vi "New Star.vi"(8 "error in (no error)":errorcluster, 10 "Board Game in":refnum<class "Board Game.lvclass">, 11 "Star in":refnum<class "Star.lvclass">) -> (0 "error out":errorcluster, 3 "Star out":refnum<class "Star.lvclass">)   [LabVIEW 2021, in "Star.lvclass"]
uses:
  Star.lvclass
  C:/Users/poche/Programs/LabVIEW/imposible snake/GameEl_class/GameEl.lvclass
  Board Game_class/Board Game.lvclass
  GameEl_class/GameEl.lvclass/GameEl.ctl
  Board Game_class/Board Game.lvclass/Board Game.ctl
  Star.lvclass/Star.ctl
  Board Game_class/Read Size.vi
  GameEl_class/GameEl.lvclass
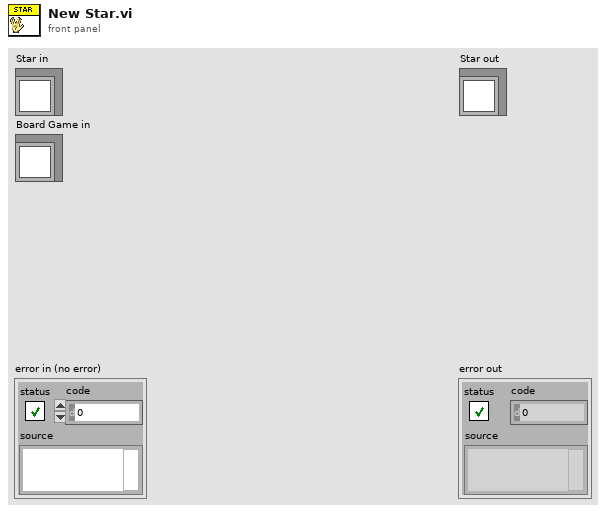
[diagram p1: front panel]
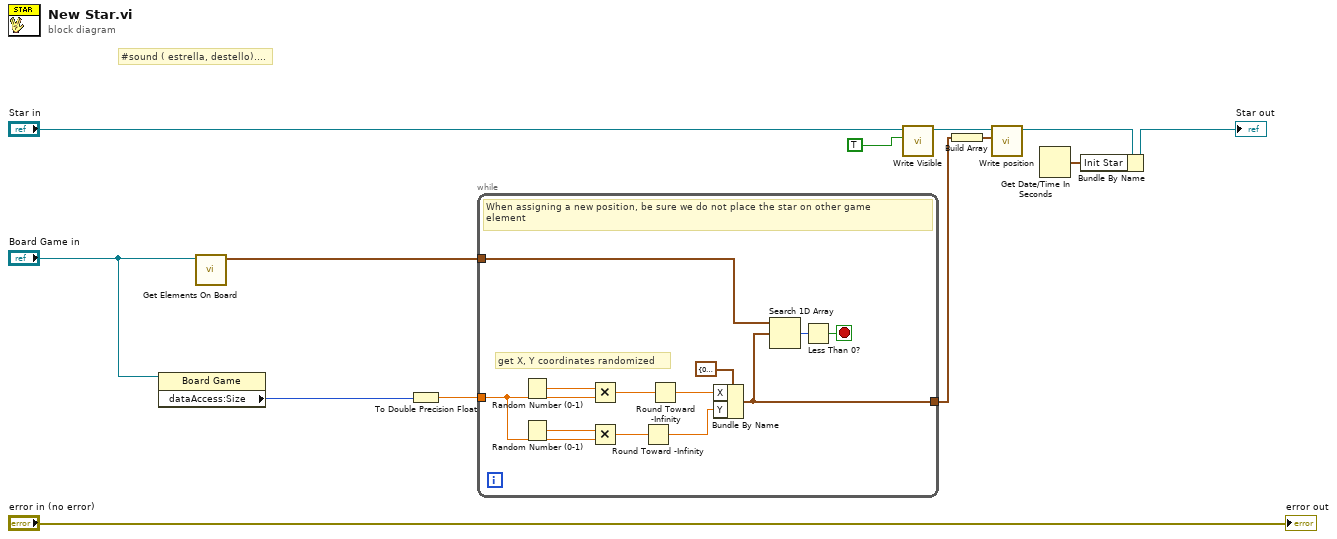
[diagram p0: block diagram]
diagram:
  # "#sound ( estrella, destello)...."
  n1 = property class="Board Game"(reference="Board Game in") -> ("dataAccess:Size"=w10:u16)  [unwired: 1 in, 2 out]
  n2 = call "Get Elements On Board.vi"("Board Game in"="Board Game in") -> ("position"=w2:cluster{"x":dbl, "y":dbl}[])  [unwired: 9 in, 1 out]
  n3 = To Double Precision Float(number=w10) -> (double precision float=w8:dbl)
  n4 = while {
    tunnel: w8 -> [w23]
    tunnel: [w16] -> w5
    tunnel: w2 -> [w15]
    stop <- w14 stop-if-true
    # "get X, Y coordinates randomized"
    # "When assigning a new position, be sure we do not place the star on other game \nelement"
    n5 = Random Number (0-1)() -> (number: 0 to 1=w25:dbl)
    n6 = Random Number (0-1)() -> (number: 0 to 1=w24:dbl)
    n7 = Multiply(x=w25, y=w23) -> (x*y=w21:dbl)
    n8 = Multiply(x=w24, y=w23) -> (x*y=w20:dbl)
    n9 = Round Toward -Infinity(1:w20) -> (0:w17:dbl)
    n10 = Round Toward -Infinity(1:w21) -> (0:w18:dbl)
    n11 = Bundle By Name(cluster=cluster{"X":dbl, "Y":dbl} {"X"=0.0, "Y"=0.0} ("Position"), "X"=w18, "Y"=w17) -> (w16:cluster{"X":dbl, "Y":dbl})
    n12 = Search 1D Array(1D array=w15, element=w16) -> (index of element=w19:i32)  [unwired: 1 in]
    n13 = Less Than 0?(x=w19) -> (x < 0?=w14:bool)
  }
  n14 = call "Write Visible.vi"("Visible"=TRUE, "GameEl in"="Star in") -> ("GameEl out"=w7:refnum<class "Star.lvclass">)  [unwired: 8 in, 1 out]
  n15 = Build Array(w5) -> (w4:cluster{"X":dbl, "Y":dbl}[])
  n16 = call "Write position.vi"("position"=w4, "GameEl in"=w7) -> ("GameEl out"=w6:refnum<class "Star.lvclass">)  [unwired: 8 in, 1 out]
  n17 = Get Date/Time In Seconds() -> (seconds since 1Jan1904=w9:timestamp)
  n18 = Bundle By Name(cluster=w6, "Init Star"=w9) -> (→"Star out":refnum<class "Star.lvclass">)
  "error out" <- "error in (no error)"
